vi "MCSA_Main[FPGA].vi"() -> ()   [LabVIEW 2017]
uses:
  <vilib>/rvi/DataTransferAndStorage/Container/XNode/niFpgaContainer.xnode
  <vilib>/eio/EIONode/EIONode.xnode
  <vilib>/addons/InsightCM/Devices/Shared/Mcsa/Fpga/McsaAcquire/subVIs/McsaAPI/MCSA_API.lvlib
  <vilib>/rvi/eio/common/nirviEmuTemplateMethod_errors.vi
  <vilib>/rvi/interface/RandomDataEmulation/nirviRandomDataFpgaReadWriteTemplate.vi
panel:
  in  "delta connection? (F)":bool
  out "FPGA Error":errorcluster
  out "Finished":bool
  in  "Stop":bool
  out "Module Underflow":bool
  out "DMA FIFO Full":bool
  out "Chan Count":bool
  out "Acq Loop Ticks":u32
  out "Chassis Temperature":sgl
  out "First Read":bool
  in  "Total Avail Channels":i32=4
  in  "Data Rate [S/s]":u32=1280
  in  "Custom Scale Slope":sgl[](array[numeric])=[0.0, 0.0, 0.0, 0.0, 0.0, 0.0, 0.0, 0.0, 0.0, 0.0, 0.0, 0.0, 0.0, 0.0, 0.0, 0.0, 0.0, 0.0, 0.0, 0.0, 0.0, 0.0, 0.0, 0.0, 0.0, 0.0, 0.0, 0.0, 0.0, 0.0, 0.0]
  in  "Acquisition Type":enum16{"Finite Samples", "Continuous Samples"}(ring)
  in  "Samps per Chan [Finite]":i32=5120
  in  "Number of Modules":i16=1
  in  "Enable Chan Array":bool[](array[boolean])=[FALSE, FALSE, FALSE, FALSE, FALSE, FALSE, FALSE, FALSE, FALSE, FALSE, FALSE, FALSE, FALSE, FALSE, FALSE, FALSE, FALSE, FALSE, FALSE, FALSE, FALSE, FALSE, FALSE, FALSE, FALSE, FALSE, FALSE, FALSE, FALSE, FALSE, FALSE]
  in  "Custom Scale Intercept":sgl[](array[numeric])=[0.0, 0.0, 0.0, 0.0, 0.0, 0.0, 0.0, 0.0, 0.0, 0.0, 0.0, 0.0, 0.0, 0.0, 0.0, 0.0, 0.0, 0.0, 0.0, 0.0, 0.0, 0.0, 0.0, 0.0, 0.0, 0.0, 0.0, 0.0, 0.0, 0.0, 0.0]
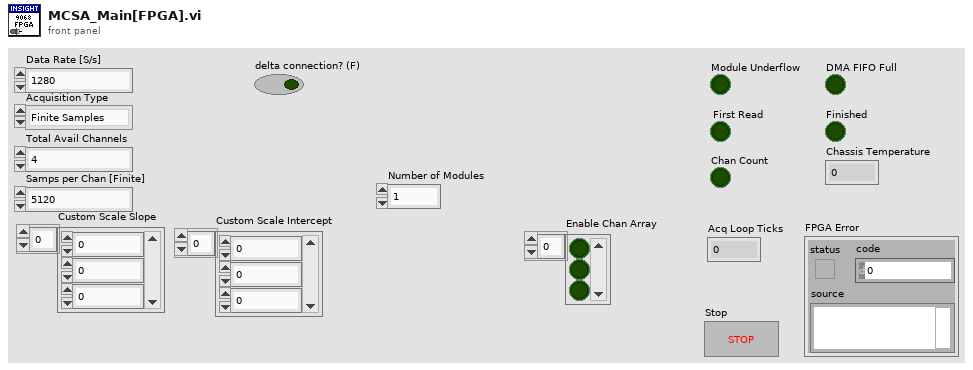
[diagram p1: front panel]
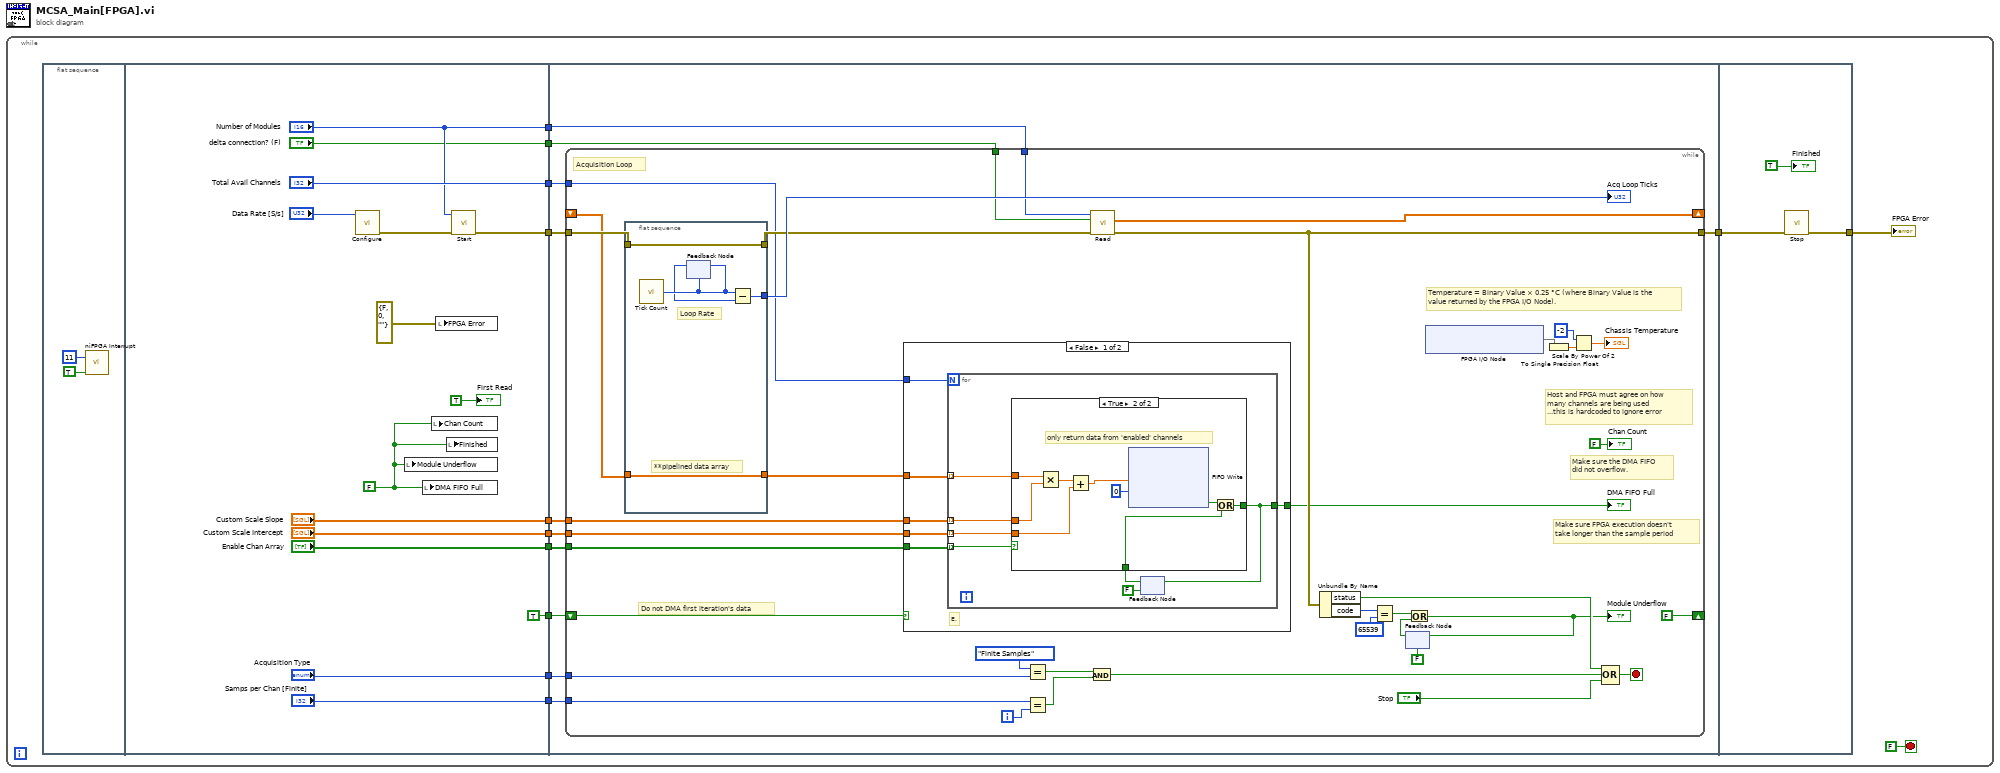
[diagram p0: block diagram]
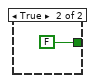
[diagram p3: hidden frame]
diagram:
  n1 = while {
    stop <- FALSE stop-if-true
    n2 = flat-sequence {
      tunnel: [w23] -> w12
      tunnel: ["Custom Scale Slope"] -> w11
      tunnel: ["Acquisition Type"] -> w10
      tunnel: ["Samps per Chan [Finite]"] -> w9
      tunnel: ["Total Avail Channels"] -> w8
      tunnel: [TRUE ("t")] -> w7
      tunnel: ["Number of Modules"] -> w5
      tunnel: ["Enable Chan Array"] -> w4
      tunnel: ["Custom Scale Intercept"] -> w2
      tunnel: ["delta connection? (F)"] -> w1
      tunnel: w12 -> [w40]
      tunnel: w11 -> [w39]
      tunnel: w10 -> [w37]
      tunnel: w9 -> [w36]
      tunnel: w8 -> [w41]
      tunnel: w7 -> [w38]
      tunnel: [w35] -> w6
      tunnel: w5 -> [w34]
      tunnel: w4 -> [w33]
      tunnel: w2 -> [w32]
      tunnel: w1 -> [w31]
      tunnel: w6 -> [w109]
      tunnel: [w108] -> w3
      frame #0 {
        n3 = call <vilib>:"niFPGA Interrupt.vi"("Wait Until Cleared (F)"=TRUE ("Wait Until Cleared"), "IRQ Number (0)"=u8 11 ("IRQ Number")) -> ()  [unwired: 1 in]
      }
      frame #1 {
        w24 = FALSE ("Module Underflow")
        n4 = call <vilib>:"Configure.vi"("Data Rate [S/s]"="Data Rate [S/s]") -> ("error out"=w21:errorcluster)  [unwired: 10 in]
        n5 = local write "Module Underflow"(w24) -> ()
        n6 = local write "DMA FIFO Full"(w24) -> ()
        n7 = local write "Chan Count"(w24) -> ()
        n8 = local write "FPGA Error"(errorcluster {"status"=FALSE, "code"=0, "source"=""} ("FPGA Error")) -> ()
        n9 = local write "Finished"(w24) -> ()
        n10 = call <vilib>:"Start.vi"("error in (no error)"=w21, "number of modules"="Number of Modules") -> ("error out"=w23:errorcluster)  [unwired: 9 in]
        "First Read" <- TRUE ("First Read")
      }
      frame #2 {
        n11 = while {
          tunnel: w40 -> [w71]
          tunnel: [w72] -> w35
          tunnel: w37 -> [w74]
          tunnel: w36 -> [w73]
          shift-right: [w66] -> _
          shift-left: _ -> [w69]
          tunnel: w41 -> [w50]
          tunnel: w39 -> [w49]
          shift-right: [FALSE ("t")] -> _
          shift-left: w38 -> [w53]
          tunnel: w34 -> [w56]
          tunnel: w33 -> [w48]
          tunnel: w32 -> [w47]
          tunnel: w31 -> [w42]
          i -> [w67]
          stop <- w77 stop-if-true
          # "Temperature = Binary Value × 0.25 °C (where Binary Value is the value returned by the FPGA I/O Node)."
          # "Do not DMA first iteration's data"
          # "Acquisition Loop"
          # "Host and FPGA must agree on how \nmany channels are being used\n...this is hardcoded to ignore error"
          # "Make sure the DMA FIFO\ndid not overflow."
          # "Make sure FPGA execution doesn't\ntake longer than the sample period"
          n12 = flat-sequence {
            tunnel: [w107] -> w54
            tunnel: w71 -> [w107]
            tunnel: [w104] -> w70
            tunnel: w69 -> [w103]
            tunnel: [w103] -> w51
            frame #0 {
              # "**pipelined data array"
              # "Loop Rate"
              n13 = call "Tick Count"() -> ("Tick Count(Ticks)"=w106:u32)
              n14 = feedback-in #1(w106) -> ()
              n15 = feedback #1(w106) -> (w105:u32)
              n16 = Subtract(x=w106, y=w105) -> (x-y=w104:u32)
            }
          }
          n17 = case shown="False" w53 {
            tunnel: [w84 FALSE] -> w52
            tunnel: w49 -> [w83 _]
            tunnel: w51 -> [w82 _]
            tunnel: w50 -> [w81 _]
            tunnel: w48 -> [w80 _]
            tunnel: w47 -> [w79 _]
            frame False {
              # "E."
              n18 = for {
                N: w81 -> [_]
                tunnel: [w90] -> w84
                tunnel: w82 -> [w89] mode=indexing
                tunnel: w83 -> [w88] mode=indexing
                tunnel: w80 -> [w86] mode=indexing
                tunnel: w79 -> [w85] mode=indexing
                n19 = feedback #2(FALSE) -> (w91:bool)
                n20 = case shown="True" w86 {
                  tunnel: w91 -> [w92 w101]
                  tunnel: [w92 w100] -> w90
                  tunnel: w89 -> [_ w99]
                  tunnel: w88 -> [_ w98]
                  tunnel: w85 -> [_ w93]
                  frame False {
                  }
                  frame True {
                    # "only return data from 'enabled' channels"
                    n21 = Multiply(x=w99, y=w98) -> (x*y=w95:sgl)
                    n22 = Add(x=w95, y=w93) -> (x+y=w94:sgl)
                    n23 = xnode ("FIFO Write")("Element"=w94, "Timeout"=0) -> ("Timed Out?"=w96:bool)  [unwired: 1 in, 1 out]
                    n24 = Or(x=w96, y=w101) -> (x .or. y?=w100:bool)
                  }
                }
                n25 = feedback-in #2(w90) -> ()
              }
            }
            frame True {
            }
          }
          "DMA FIFO Full" <- w52
          n26 = Equal?(x=enum16{"Finite Samples", "Continuous Samples"}."Finite Samples" ("y"), y=w74) -> (x = y?=w60:bool)
          n27 = Equal?(x=w73, y=w67) -> (x = y?=w59:bool)
          n28 = And(x=w60, y=w59) -> (x .and. y?=w58:bool)
          n29 = call <vilib>:"Read.vi"("error in (no error)"=w54, "delta connection? (F)"=w42, "number of modules"=w56) -> ("error out"=w72:errorcluster, "Data Array"=w66:sgl[])  [unwired: 7 in]
          n30 = Unbundle By Name(w72) -> ("status"=w65:bool, "code"=w75:i32)
          n31 = Equal?(x=w75, y=65539) -> (x = y?=w62:bool)
          n32 = feedback #3(FALSE) -> (w64:bool)
          n33 = Or(x=w62, y=w64) -> (x .or. y?=w61:bool)
          "Module Underflow" <- w61
          n34 = feedback-in #3(w61) -> ()
          n35 = xnode "FPGA I/O Node"() -> ("Chassis Temperature"=w44)  [unwired: 1 in, 1 out]
          n36 = To Single Precision Float(number=w44) -> (single precision float=w46:sgl)
          n37 = Scale By Power Of 2(n=i16 -2, x=w46) -> (x*2^n=→"Chassis Temperature":sgl)
          n38 = Compound Arithmetic op=OR(w65, w58, "Stop") -> (w77:bool)
          "Chan Count" <- FALSE ("Chan Count")
          "Acq Loop Ticks" <- w70
        }
      }
      frame #3 {
        n39 = call <vilib>:"Stop.vi"("error in (no error)"=w109) -> ("error out"=w108:errorcluster)  [unwired: 10 in]
        "Finished" <- TRUE ("Finished")
      }
    }
    "FPGA Error" <- w3
  }
